vi "Delete Global.vi"(8 "error in (no error)":errorcluster) -> (0 "error out":errorcluster)   [LabVIEW 2019, in "GaitDAQ UI.lvlib"]
uses:
  GaitDAQ UI.lvlib
  <userlib>/JUL/Event Message Module/Event Message Library/Event Message.lvlib
panel:
  # "Input"
  # "Output"
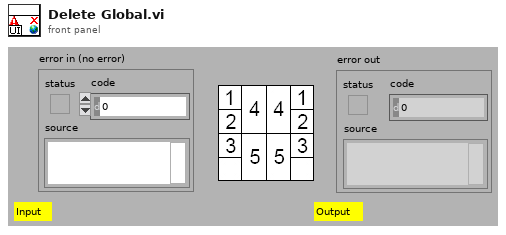
[diagram p1: front panel]
types:
  T1 = typedef "GaitDAQ UI.lvlib/Event Registration Refnum.ctl" = refnum<event-registration>
  T2 = typedef "Event Message.lvlib/Event.ctl" = refnum<user-event>
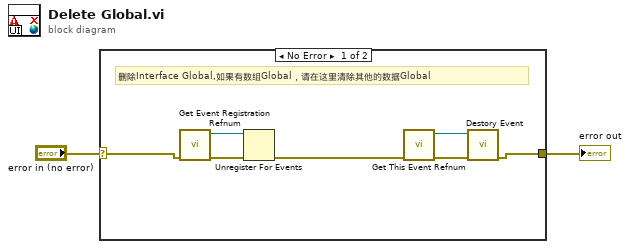
[diagram p0: block diagram]
diagram:
  n1 = case shown="No Error" "error in (no error)" {
    selector: "error in (no error)" -> [w6 w10]
    tunnel: [w8 w10] -> w1
    frame No Error {
      # "删除Interface Global,如果有数组Global，请在这里清除其他的数据Global"
      n2 = call "Get Event Registration Refnum.vi"("error in (no error)"=w6) -> ("error out"=w5:errorcluster, "Event Registration Refnum out"=w4:T1)  [unwired: 9 in]
      n3 = Unregister For Events(event registration refnum=w4, error in=w5) -> (error out=w3:errorcluster)
      n4 = call "Get This Event Refnum.vi"("error in (no error)"=w3) -> ("error out"=w7:errorcluster, "This Event Refnum Out"=w9:T2)  [unwired: 9 in]
      n5 = call <userlib>:"Destory Event.vi"("error in (no error)"=w7, "Event In"=w9) -> ("error out"=w8:errorcluster)  [unwired: 9 in]
    }
    frame Error {
    }
  }
  "error out" <- w1
